vi "SerialFWDR2.vi"(8 "error in (no error)":errorcluster, 9 "Delay Time (s)":dbl=1.0, 10 "CommandString":string, 11 "VISA Refnum in":refnum<visa-resource-name>) -> (0 "error out":errorcluster, 2 "trimmed string":string, 3 "VISA Refnum out":refnum<visa-resource-name>)   [LabVIEW 2017]
uses:
  <vilib>/Instr/_visa.llb/VISA Flush IO Buffer Mask.ctl
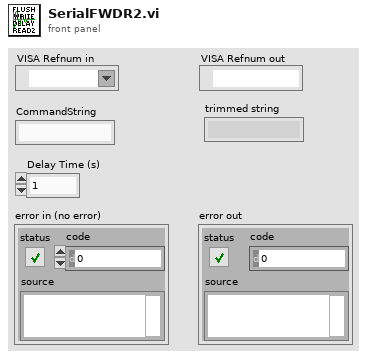
[diagram p1: front panel]
types:
  T1 = typedef "VISA Flush IO Buffer Mask.ctl" = u16
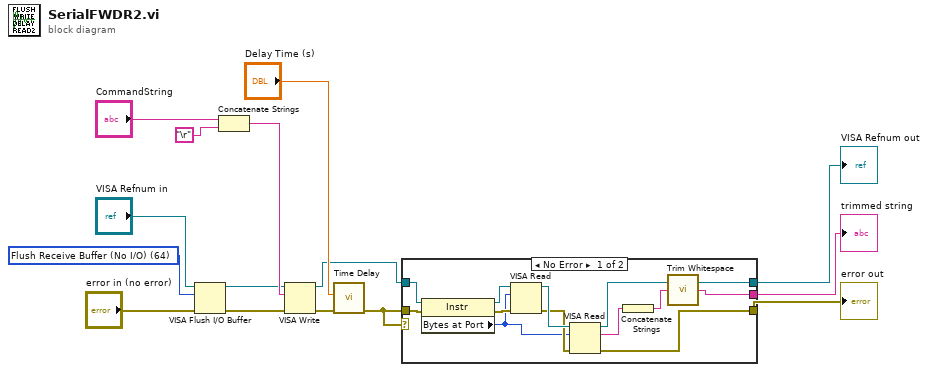
[diagram p0: block diagram]
diagram:
  w9 = T1 64 items=["Flush Receive Buffer"=16, "Write Transmit Buffer to Device"=32, "Flush Receive Buffer (No I/O)"=64, "Flush Transmit Buffer"=128] ("Mask")
  n1 = VISA Flush I/O Buffer(VISA resource name="VISA Refnum in", mask (16)=w9, error in (no error)="error in (no error)") -> (VISA resource name out=w3:refnum<visa-resource-name>, error out=w2:errorcluster)
  n2 = Concatenate Strings("CommandString", "\r") -> (w12:string)
  n3 = VISA Write(VISA resource name=w3, write buffer=w12, error in (no error)=w2) -> (VISA resource name out=w8:refnum<visa-resource-name>, error out=w10:errorcluster)  [unwired: 1 out]
  n4 = call "Time Delay"("error in (no error)"=w10, "Delay Time (s)"="Delay Time (s)") -> ("error out"=w4:errorcluster)  [unwired: 9 in]
  n5 = case shown="No Error" w4 {
    tunnel: w4 -> [w26 w29]
    tunnel: [w20 w29] -> w7
    tunnel: [w22 w28] -> w5
    tunnel: w8 -> [w24 w28]
    tunnel: [w18 _] -> w6
    frame No Error {
      n6 = property class="Instr"(reference=w24, error in=w26) -> (reference out=w27:refnum<visa-resource-name>, error out=w25:errorcluster, "Bytes at Port"=w16:u32)
      n7 = VISA Read(VISA resource name=w27, byte count=w16, error in (no error)=w25) -> (VISA resource name out=w23:refnum<visa-resource-name>, error out=w21:errorcluster)  [unwired: 2 out]
      n8 = VISA Read(VISA resource name=w23, byte count=w16, error in (no error)=w21) -> (VISA resource name out=w22:refnum<visa-resource-name>, read buffer=w19:string, error out=w20:errorcluster)  [unwired: 1 out]
      n9 = Concatenate Strings(w19) -> (w17:string)
      n10 = call <vilib>:"Trim Whitespace.vi"("string"=w17) -> ("trimmed string"=w18:string)  [unwired: 1 in]
    }
    frame Error {
    }
  }
  "VISA Refnum out" <- w5
  "error out" <- w7
  "trimmed string" <- w6
